vi "Exit Phase.vi"(8 "error in (no error)":errorcluster, 11 "Programming Logicv2 in":refnum<class "Programming Logicv2.lvclass">) -> (0 "error out":errorcluster, 3 "Programming Logicv2 out":refnum<class "Programming Logicv2.lvclass">)   [LabVIEW 2014, in "Main Libraryv2.lvlib" / "Programming Logicv2.lvclass"]
uses:
  Programming Logicv2.lvclass
  <vilib>/NI/Modbus Library/API/Master/Modbus Master.lvclass
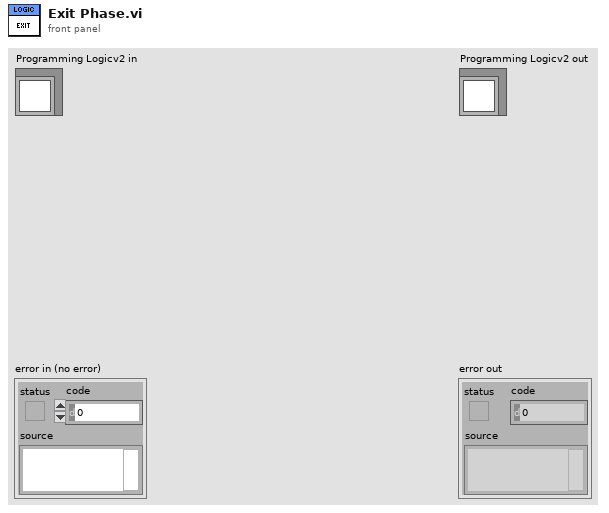
[diagram p1: front panel]
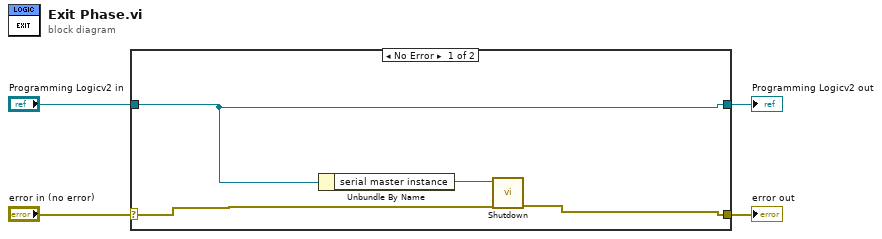
[diagram p0: block diagram]
diagram:
  n1 = case shown="No Error" "error in (no error)" {
    selector: "error in (no error)" -> [w7 w10]
    tunnel: [w6 w10] -> w3
    tunnel: [w5 w9] -> w1
    tunnel: "Programming Logicv2 in" -> [w5 w9]
    frame No Error {
      n2 = Unbundle By Name(w5) -> ("serial master instance"=w8:refnum<class "Modbus Master.lvclass">)
      n3 = call-dynamic "Shutdown.vi"("error in"=w7, "Modbus master in"=w8) -> ("error out"=w6:errorcluster)  [unwired: 9 in]
    }
    frame Error {
    }
  }
  "error out" <- w3
  "Programming Logicv2 out" <- w1
